vi "GetListing.vi"(9 "path":string, 10 "Ftp":refnum<k24>, 11 "error in":errorcluster) -> (1 "Items":T1(array[cluster]), 3 "error out":errorcluster)   [LabVIEW 2019, in "UnderAutomation.Fanuc.lvlib"]
uses:
  UnderAutomation.Fanuc.lvlib
  C:/Users/fg/Documents/Fanuc.vi/LabVIEW_2024/UnderAutomation.Fanuc/lib/UnderAutomation.Fanuc.dll
  LabVIEW_2024/UnderAutomation.Fanuc/lib/UnderAutomation.Fanuc.dll
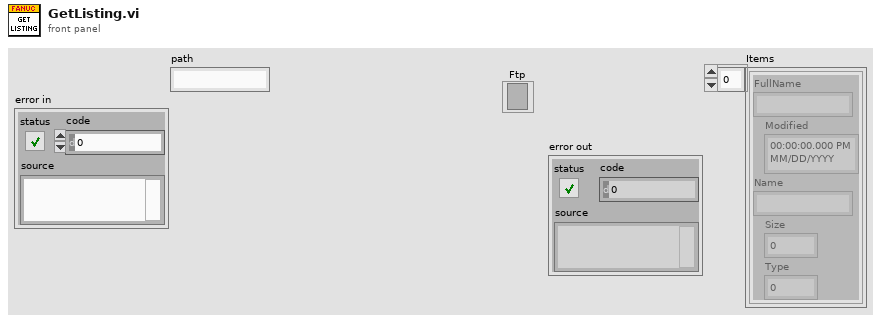
[diagram p1: front panel]
types:
  T1 = cluster{"FullName":string, "Modified":timestamp, "Name":string, "Size":i64, "Type":i32}[]
  T2 = cluster{"FullName":string, "Modified":timestamp, "Name":string, "Size":i64, "Type":i32}
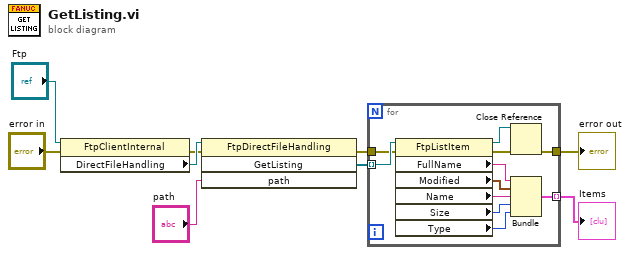
[diagram p0: block diagram]
diagram:
  n1 = property class="FtpClientInternal"(reference="Ftp", error in="error in") -> (error out=w5:errorcluster, "DirectFileHandling"=w7:refnum<k24>)  [unwired: 1 out]
  n2 = invoke class="FtpDirectFileHandling" method="GetListing"(reference=w7, error in=w5, "path"="path") -> (error out=w2:errorcluster, "GetListing"=w4:refnum<k24>[])  [unwired: 1 in, 2 out]
  n3 = for {
    tunnel: w4 -> [w20] mode=indexing
    tunnel: [w14] -> w3 mode=indexing
    tunnel: w2 -> [w13]
    tunnel: [w10] -> w1
    n4 = property class="FtpListItem"(reference=w20, error in=w13) -> (reference out=w11:refnum<k24>, error out=w12:errorcluster, "FullName"=w19:string, "Modified"=w18:timestamp, "Name"=w17:string, "Size"=w16:i64, "Type"=w15:i32)
    n5 = Close Reference(reference=w11, error in (no error)=w12) -> (error out=w10:errorcluster)
    n6 = Bundle("FullName"=w19, "Modified"=w18, "Name"=w17, "Size"=w16, "Type"=w15) -> (w14:T2)  [unwired: 1 in]
  }
  "error out" <- w1
  "Items" <- w3
